vi "Sensor Loop.vi"() -> ()   [LabVIEW 2017]
uses:
  <vilib>/Platform/TimedLoop/XDataNode/timing_clust.ctl
  <vilib>/Platform/TimedLoop/XDataNode/nitl_modes.ctl
  <vilib>/Platform/TimedLoop/XDataNode/wakeup.ctl
  <vilib>/Rock Robotics/Network Tables/NT Read Number.vi
  <vilib>/platform/TimedLoop/XDataNode/XDataNode.xnode
  <vilib>/Platform/TimedLoop/XDataNode/XDNodeRunTimeDep.lvlib
panel:
  in  "Period":i64
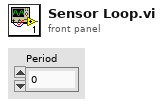
[diagram p1: front panel]
types:
  T1 = typedef "WPI_AnalogChannelDevRef.ctl" = cluster{"DevStatus":errorcluster, "Analog Channel":T2}
  T2 = typedef "FPGA_AIChannel.ctl" = enum8{"AI 0", "AI 1", "AI 2", "AI 3", "AI MXP 0", "AI MXP 1", "AI MXP 2", "AI MXP 3", "Invalid"}
  T3 = typedef "WPI_DigitalInputDevRef.ctl" = cluster{"DevStatus":errorcluster, "DIO Channel":T4}
  T4 = typedef "FPGA_DIOChannel.ctl" = enum8{"DIO 0", "DIO 1", "DIO 2", "DIO 3", "DIO 4", "DIO 5", "DIO 6", "DIO 7", "DIO 8", "DIO 9", "DIO MXP 0", "DIO MXP 1", "DIO MXP 2", "DIO MXP 3", "DIO MXP 4", "DIO MXP 5", "DIO MXP 6", "DIO MXP 7", "DIO MXP 8", "DIO MXP 9", "DIO MXP 10", "DIO MXP 11", "DIO MXP 12", "DIO MXP 13", "DIO MXP 14", "DIO MXP 15", "SPI Port CS1", "SPI Port CS2", "SPI Port CS3", "SPI Port MISO", "SPI Port MOSI", "Invalid"}
  T5 = typedef "WPI_EncoderDevRef.ctl" = cluster{"DevStatus":errorcluster, "EncoderIndex":T6, "CounterIndex":T7, "DistancePerCount":dbl, "Decoding Type":T8}
  T6 = typedef "FPGA_EncoderIdx.ctl" = enum8{"Enc 0", "Enc 1", "Enc 2", "Enc 3", "Enc 4", "Enc 5", "Enc 6", "Enc 7", "Invalid"}
  T7 = typedef "FPGA_CounterCtrSystemIndex.ctl" = enum8{"Ctr 0", "Ctr 1", "Ctr 2", "Ctr 3", "Ctr 4", "Ctr 5", "Ctr 6", "Ctr 7", "Invalid"}
  T8 = typedef "WPI_EncoderType.ctl" = enum16{"1x", "2x", "4x"}
  T9 = typedef "ImuDevRef.ctl" = cluster{"I2CDevRef":T10, "Valid Cal File?":bool}
  T10 = typedef "WPI_I2CDevRef.ctl" = cluster{"DevStatus":errorcluster, "Device Address":u8, "Handle":i32, "I2C Bus":T11}
  T11 = typedef "i2c_bus.ctl" = enum16{"I2C On-Board", "I2C MXP", "Invalid"}
  T12 = typedef "XDNodeRunTimeDep.lvlib/timing_clust.ctl" = cluster{"Expected End [f-1]":u64, "Actual End [f-1]":u64, "Finished Late? [f-1]":bool, "Expected End [i-1]":u64, "Actual End [i-1]":u64, "Finished Late? [i-1]":bool, "Expected Start [i]":u64, "Actual Start [i]":u64, "Expected Start [f]":u64, "Actual Start [f]":u64, "Source Name":string, "Structure Name":string, "Period":i64, "Deadline":i64, "Offset":i64, "Start":i64, "Priority":i32, "Timeout":i32, "Mode":T13, "Wakeup Reason":T14, "Error":errorcluster, "Source Type":string, "Secondary Source Type":string, "Global End Time":u64, "Global Start Time":u64, "Frame Duration":u64, "Iteration Duration":u64, "Assigned CPU":i32, "I/O Scan Engine Mode":u32}
  T13 = typedef "XDNodeRunTimeDep.lvlib/nitl_modes.ctl" = enum32{"No Change", "Process missed periods, maintain original phase", "Discard missed periods, maintain original phase", "Process missed periods, ignore original phase", "Discard missed periods, ignore original phase"}
  T14 = typedef "XDNodeRunTimeDep.lvlib/wakeup.ctl" = enum32{"Normal", "Aborted", "Asynchronous wakeup", "Timing source error", "Timed loop error", "Timeout"}
  T15 = cluster{"Yaw":dbl, "Roll":dbl, "Pitch":dbl, "Yaw Wind":dbl, "Roll Wind":dbl, "Pitch Wind":dbl}
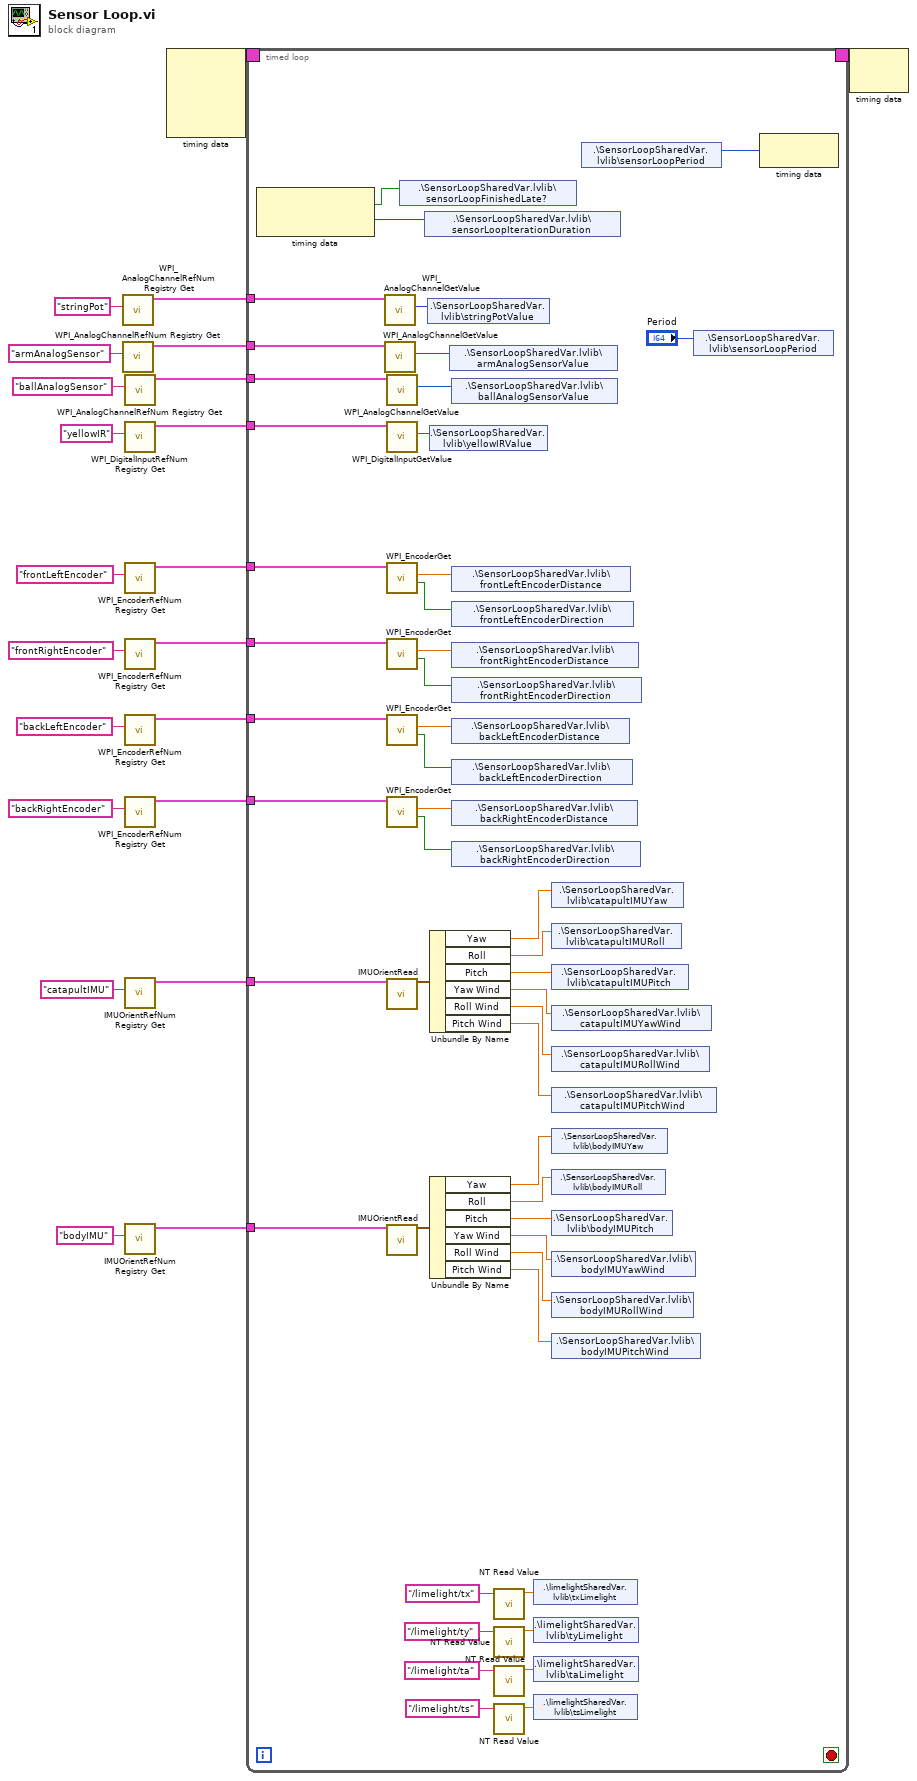
[diagram p0: block diagram]
diagram:
  n1 = call <vilib>:"WPI_AnalogChannelRefNum Registry Get.vi"("refnum name"="stringPot") -> ("AIDeviceRef"=w3:T1)  [unwired: 9 in, 1 out]
  n2 = call <vilib>:"WPI_AnalogChannelRefNum Registry Get.vi"("refnum name"="armAnalogSensor") -> ("AIDeviceRef"=w4:T1)  [unwired: 9 in, 1 out]
  n3 = call <vilib>:"WPI_AnalogChannelRefNum Registry Get.vi"("refnum name"="ballAnalogSensor") -> ("AIDeviceRef"=w5:T1)  [unwired: 9 in, 1 out]
  n4 = call <vilib>:"WPI_DigitalInputRefNum Registry Get.vi"("refnum name"="yellowIR") -> ("DigitalInputDevRef"=w1:T3)  [unwired: 9 in, 1 out]
  n5 = call <vilib>:"WPI_EncoderRefNum Registry Get.vi"("refnum name"="frontLeftEncoder") -> ("EncoderDevRef"=w13:T5)  [unwired: 9 in, 1 out]
  n6 = call <vilib>:"WPI_EncoderRefNum Registry Get.vi"("refnum name"="frontRightEncoder") -> ("EncoderDevRef"=w15:T5)  [unwired: 9 in, 1 out]
  n7 = call <vilib>:"WPI_EncoderRefNum Registry Get.vi"("refnum name"="backLeftEncoder") -> ("EncoderDevRef"=w17:T5)  [unwired: 9 in, 1 out]
  n8 = call <vilib>:"WPI_EncoderRefNum Registry Get.vi"("refnum name"="backRightEncoder") -> ("EncoderDevRef"=w19:T5)  [unwired: 9 in, 1 out]
  n9 = call <userlib>:"IMUOrientRefNum Registry Get.vi"("refnum name"="catapultIMU") -> ("IMUDevRef out"=w9:T9)  [unwired: 9 in, 1 out]
  n10 = call <userlib>:"IMUOrientRefNum Registry Get.vi"("refnum name"="bodyIMU") -> ("IMUDevRef out"=w10:T9)  [unwired: 9 in, 1 out]
  n11 = node-c288() -> (w22:T12)  [unwired: 4 in]
  n12 = timed-loop {
    timing: w22 -> [_]
    timing-out: [_] -> w21
    tunnel: w19 -> [w70]
    tunnel: w17 -> [w67]
    tunnel: w15 -> [w64]
    tunnel: w13 -> [w61]
    tunnel: w10 -> [w58]
    tunnel: w9 -> [w57]
    tunnel: w5 -> [w42]
    tunnel: w4 -> [w41]
    tunnel: w3 -> [w40]
    tunnel: w1 -> [w36]
    stop <- _ stop-if-true
    n13 = node-c288() -> (w33:bool, w34:i64)  [unwired: 1 in]
    n14 = call <vilib>:"WPI_AnalogChannelGetValue.vi"("AIDeviceRef"=w40) -> ("Value"=w39:i16)  [unwired: 8 in, 2 out]
    n15 = call <vilib>:"WPI_AnalogChannelGetValue.vi"("AIDeviceRef"=w41) -> ("Value"=w38:i16)  [unwired: 8 in, 2 out]
    n16 = call <vilib>:"WPI_AnalogChannelGetValue.vi"("AIDeviceRef"=w42) -> ("Value"=w37:i16)  [unwired: 8 in, 2 out]
    n17 = call <vilib>:"WPI_DigitalInputGetValue.vi"("DigitalInputDevRef"=w36) -> ("Value"=w35:bool)  [unwired: 8 in, 2 out]
    n18 = call <vilib>:"WPI_EncoderGet.vi"("EncoderDevRef"=w61) -> ("Direction"=w59:bool, "Distance"=w60:dbl)  [unwired: 5 in, 4 out]
    n19 = call <vilib>:"WPI_EncoderGet.vi"("EncoderDevRef"=w64) -> ("Direction"=w62:bool, "Distance"=w63:dbl)  [unwired: 5 in, 4 out]
    n20 = call <vilib>:"WPI_EncoderGet.vi"("EncoderDevRef"=w67) -> ("Direction"=w65:bool, "Distance"=w66:dbl)  [unwired: 5 in, 4 out]
    n21 = call <vilib>:"WPI_EncoderGet.vi"("EncoderDevRef"=w70) -> ("Direction"=w68:bool, "Distance"=w69:dbl)  [unwired: 5 in, 4 out]
    n22 = call <userlib>:"IMUOrientRead.vi"("IMU Dev Ref"=w57) -> ("Orient Y/R/P"=w55:T15)  [unwired: 7 in, 7 out]
    n23 = call <userlib>:"IMUOrientRead.vi"("IMU Dev Ref"=w58) -> ("Orient Y/R/P"=w56:T15)  [unwired: 7 in, 7 out]
    n24 = shared-variable ".\\SensorLoopSharedVar.lvlib\\sensorLoopFinishedLate?"(w33) -> ()  [unwired: 1 in, 1 out]
    n25 = shared-variable ".\\SensorLoopSharedVar.lvlib\\sensorLoopIterationDuration"(w34) -> ()  [unwired: 1 in, 1 out]
    n26 = shared-variable ".\\SensorLoopSharedVar.lvlib\\stringPotValue"(w39) -> ()  [unwired: 1 in, 1 out]
    n27 = shared-variable ".\\SensorLoopSharedVar.lvlib\\yellowIRValue"(w35) -> ()  [unwired: 1 in, 1 out]
    n28 = Unbundle By Name(w55) -> ("Yaw"=w48:dbl, "Roll"=w47:dbl, "Pitch"=w46:dbl, "Yaw Wind"=w45:dbl, "Roll Wind"=w44:dbl, "Pitch Wind"=w43:dbl)
    n29 = Unbundle By Name(w56) -> ("Yaw"=w54:dbl, "Roll"=w53:dbl, "Pitch"=w52:dbl, "Yaw Wind"=w51:dbl, "Roll Wind"=w50:dbl, "Pitch Wind"=w49:dbl)
    n30 = shared-variable ".\\SensorLoopSharedVar.lvlib\\armAnalogSensorValue"(w38) -> ()  [unwired: 1 in, 1 out]
    n31 = shared-variable ".\\SensorLoopSharedVar.lvlib\\ballAnalogSensorValue"(w37) -> ()  [unwired: 1 in, 1 out]
    n32 = shared-variable ".\\SensorLoopSharedVar.lvlib\\frontLeftEncoderDistance"(w60) -> ()  [unwired: 1 in, 1 out]
    n33 = shared-variable ".\\SensorLoopSharedVar.lvlib\\frontLeftEncoderDirection"(w59) -> ()  [unwired: 1 in, 1 out]
    n34 = shared-variable ".\\SensorLoopSharedVar.lvlib\\frontRightEncoderDistance"(w63) -> ()  [unwired: 1 in, 1 out]
    n35 = shared-variable ".\\SensorLoopSharedVar.lvlib\\frontRightEncoderDirection"(w62) -> ()  [unwired: 1 in, 1 out]
    n36 = shared-variable ".\\SensorLoopSharedVar.lvlib\\backLeftEncoderDistance"(w66) -> ()  [unwired: 1 in, 1 out]
    n37 = shared-variable ".\\SensorLoopSharedVar.lvlib\\backLeftEncoderDirection"(w65) -> ()  [unwired: 1 in, 1 out]
    n38 = shared-variable ".\\SensorLoopSharedVar.lvlib\\backRightEncoderDistance"(w69) -> ()  [unwired: 1 in, 1 out]
    n39 = shared-variable ".\\SensorLoopSharedVar.lvlib\\backRightEncoderDirection"(w68) -> ()  [unwired: 1 in, 1 out]
    n40 = call-poly <vilib>:"NT Read Value.vi"("Name"="/limelight/tx") -> ("Numeric"=w26:dbl)  [unwired: 9 in, 1 out]
    n41 = call-poly <vilib>:"NT Read Value.vi"("Name"="/limelight/ty") -> ("Numeric"=w25:dbl)  [unwired: 9 in, 1 out]
    n42 = call-poly <vilib>:"NT Read Value.vi"("Name"="/limelight/ta") -> ("Numeric"=w24:dbl)  [unwired: 9 in, 1 out]
    n43 = call-poly <vilib>:"NT Read Value.vi"("Name"="/limelight/ts") -> ("Numeric"=w23:dbl)  [unwired: 9 in, 1 out]
    n44 = shared-variable ".\\limelightSharedVar.lvlib\\txLimelight"(w26) -> ()  [unwired: 1 in, 1 out]
    n45 = shared-variable ".\\limelightSharedVar.lvlib\\tyLimelight"(w25) -> ()  [unwired: 1 in, 1 out]
    n46 = shared-variable ".\\limelightSharedVar.lvlib\\taLimelight"(w24) -> ()  [unwired: 1 in, 1 out]
    n47 = shared-variable ".\\limelightSharedVar.lvlib\\tsLimelight"(w23) -> ()  [unwired: 1 in, 1 out]
    n48 = shared-variable ".\\SensorLoopSharedVar.lvlib\\catapultIMUYaw"(w48) -> ()  [unwired: 1 in, 1 out]
    n49 = shared-variable ".\\SensorLoopSharedVar.lvlib\\catapultIMURoll"(w47) -> ()  [unwired: 1 in, 1 out]
    n50 = shared-variable ".\\SensorLoopSharedVar.lvlib\\catapultIMUPitch"(w46) -> ()  [unwired: 1 in, 1 out]
    n51 = shared-variable ".\\SensorLoopSharedVar.lvlib\\catapultIMUYawWind"(w45) -> ()  [unwired: 1 in, 1 out]
    n52 = shared-variable ".\\SensorLoopSharedVar.lvlib\\catapultIMURollWind"(w44) -> ()  [unwired: 1 in, 1 out]
    n53 = shared-variable ".\\SensorLoopSharedVar.lvlib\\catapultIMUPitchWind"(w43) -> ()  [unwired: 1 in, 1 out]
    n54 = shared-variable ".\\SensorLoopSharedVar.lvlib\\bodyIMUYaw"(w54) -> ()  [unwired: 1 in, 1 out]
    n55 = shared-variable ".\\SensorLoopSharedVar.lvlib\\bodyIMURoll"(w53) -> ()  [unwired: 1 in, 1 out]
    n56 = shared-variable ".\\SensorLoopSharedVar.lvlib\\bodyIMUPitch"(w52) -> ()  [unwired: 1 in, 1 out]
    n57 = shared-variable ".\\SensorLoopSharedVar.lvlib\\bodyIMUYawWind"(w51) -> ()  [unwired: 1 in, 1 out]
    n58 = shared-variable ".\\SensorLoopSharedVar.lvlib\\bodyIMURollWind"(w50) -> ()  [unwired: 1 in, 1 out]
    n59 = shared-variable ".\\SensorLoopSharedVar.lvlib\\bodyIMUPitchWind"(w49) -> ()  [unwired: 1 in, 1 out]
    n60 = shared-variable ".\\SensorLoopSharedVar.lvlib\\sensorLoopPeriod"() -> (w32:i64)  [unwired: 1 in, 1 out]
    n61 = shared-variable ".\\SensorLoopSharedVar.lvlib\\sensorLoopPeriod"("Period") -> ()  [unwired: 1 in, 1 out]
    n62 = node-c288(w32) -> ()  [unwired: 1 out]
  }
  n63 = node-c288(w21) -> ()  [unwired: 1 out]
